vi "Write Multiple Holding Registers.vi"(8 "error in (no error)":errorcluster, 9 "holding register values":u16[](array[numeric]), 10 "starting address":u16, 11 "Modbus master in":refnum<class "Network Master.lvclass">) -> (0 "error out":errorcluster, 3 "Modbus master out":refnum<class "Network Master.lvclass">)   [LabVIEW 2021, in "Network Master.lvclass"]
doc: "Writes values to contiguous holding registers. The maximum number of holding registers this VI can write is 123."
uses:
  Network Master.lvclass
  D:/my_projects/projects/Algorithms/Labview/21/Modbus_v121c/Network Protocol/Network Protocol.lvclass
  Modbus Data Unit/Modbus Data Unit.lvclass/Modbus Data Unit.ctl
  Network Protocol.lvclass/Network Protocol.ctl
  Network Master.lvclass/Network Master.ctl
  Modbus Data Unit/Construct PDU.vi
  Utility/U16s to Bytes.vi
  Master Function Definition/Function code mismatch error.vi
  Data Model/Error Generator.vi
  Modbus Data Unit/Deconstruct PDU.vi
  Read Transmission Data Unit.vi
  Modbus Data Unit/Modbus Data Unit.lvclass
  Transmission Data Unit/Transmission Data Unit.lvclass
  Master Function Definition/Master Function Definition.lvclass
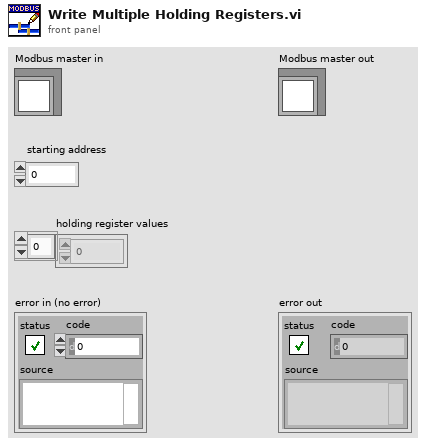
[diagram p1: front panel]
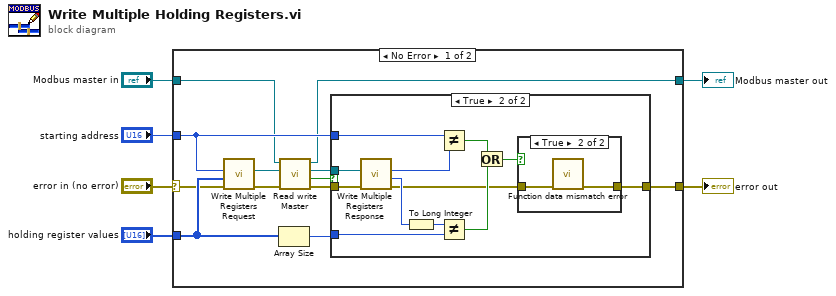
[diagram p0: block diagram]
diagram:
  n1 = case shown="No Error" "error in (no error)" {
    selector: "error in (no error)" -> [w9 w36]
    tunnel: "Modbus master in" -> [w7 w35]
    tunnel: [w17 w36] -> w3
    tunnel: [w8 w35] -> w4
    tunnel: "holding register values" -> [w14 _]
    tunnel: "starting address" -> [w16 _]
    frame No Error {
      n2 = call "Write Multiple Registers Request.vi"("error in"=w9, "Registers"=w14, "Starting Address"=w16) -> ("error out"=w18:errorcluster, "modbus data unit out"=w10:refnum<class "Modbus Data Unit.lvclass">)  [unwired: 7 in]
      n3 = Array Size(array=w14) -> (size(s)=w15:i32)
      n4 = call "Read write Master.vi"("error in (no error)"=w18, "Modbus data unit in"=w10, "Modbus master in"=w7) -> ("error out"=w13:errorcluster, "PDU valid?"=w12:bool, "Modbus data unit out"=w11:refnum<class "Modbus Data Unit.lvclass">, "Modbus master out"=w8:refnum<class "Network Master.lvclass">)  [unwired: 5 in]
      n5 = case shown="True" w12 {
        tunnel: [w19 w28] -> w17
        tunnel: w16 -> [_ w21]
        tunnel: w15 -> [_ w26]
        tunnel: w13 -> [w19 w25]
        tunnel: w11 -> [_ w24]
        frame False {
        }
        frame True {
          n6 = call "Write Multiple Registers Response.vi"("error in"=w25, "modbus data unit in"=w24) -> ("error out"=w23:errorcluster, "Number of Registers"=w27:u16, "Start Address"=w22:u16)  [unwired: 7 in]
          n7 = To Long Integer(number=w27) -> (32bit integer=w20:i32)
          n8 = Not Equal?(x=w21, y=w22) -> (x != y?=w30:bool)
          n9 = Not Equal?(x=w20, y=w26) -> (x != y?=w29:bool)
          n10 = Or(x=w30, y=w29) -> (x .or. y?=w31:bool)
          n11 = case shown="True" w31 {
            tunnel: [w32 w34] -> w28
            tunnel: w23 -> [w32 w33]
            frame False {
            }
            frame True {
              n12 = call "Function data mismatch error.vi"("error in (no error)"=w33) -> ("error out"=w34:errorcluster)  [unwired: 10 in]
            }
          }
        }
      }
    }
    frame Error {
    }
  }
  "error out" <- w3
  "Modbus master out" <- w4
